vi "Get Remote cRIO Modules Info.vi"(8 "error in":errorcluster, 9 "Device Name":string="RIO0", 10 "cRIO Backplane":T1=enum."cRIO-9068", 11 "IP Address":string) -> (0 "error out":errorcluster, 2 "cRIO Modules":T2[](array[typedef]) {"Serial Number" format="%.0x"; "Vendor and Module ID" format="%.0x"})   [LabVIEW 2015]
uses:
  Controls/cRIO Module Info.ctl
  RT Management/Controls/cRIO Backplanes.ctl
  <vilib>/FPGAPlugInAG/Dynamic/niLvFpga_Run_Dynamic.vi
  <vilib>/FPGAPlugInAG/Dynamic/niLvFpga_Close_Dynamic.vi
  <vilib>/rvi/interface/nirviMethod/nirviMethod.xnode
  <vilib>/rvi/interface/nirviCloseFPGA/nirviCloseFPGA.xnode
  Module Detection.lvclass
  RT Management/RT Management.lvclass
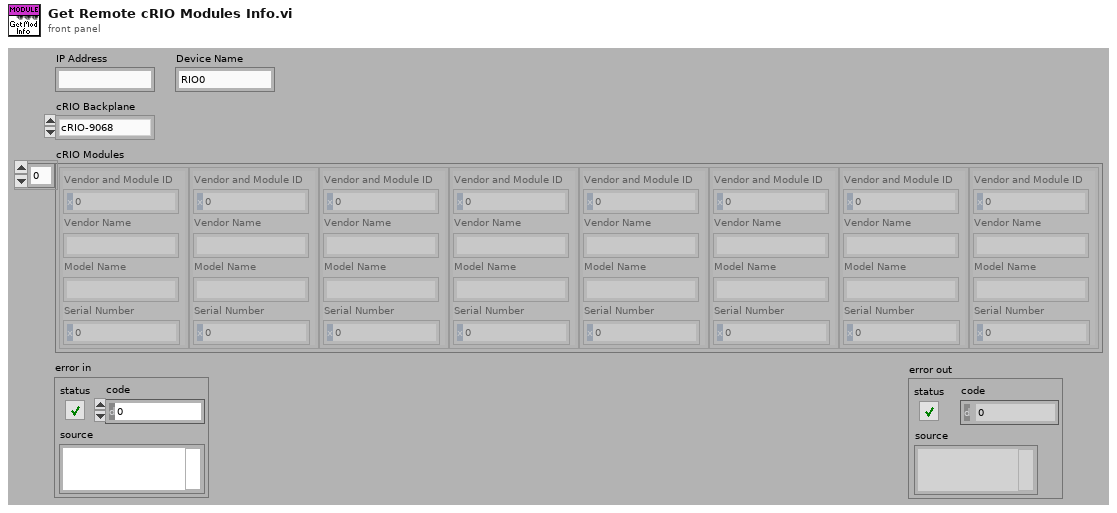
[diagram p1: front panel]
types:
  T1 = typedef "RT Management.lvlib/RT Management.lvclass/cRIO Backplanes.ctl" = enum16{"<Undefined>", "cRIO-9030", "cRIO-9031", "cRIO-9033", "cRIO-9034", "cRIO-9035", "cRIO-9036", "cRIO-9038", "cRIO-9039", "cRIO-9063", "cRIO-9064", "cRIO-9065", "cRIO-9066", "cRIO-9067", "cRIO-9068", "cRIO-9072", "cRIO-9073", "cRIO-9074", "cRIO-9075", "cRIO-9076", "cRIO-9081", "cRIO-9082", "cRIO-9101", "cRIO-9102", "cRIO-9103", "cRIO-9104", "cRIO-9111", "cRIO-9112", "cRIO-9113", "cRIO-9114", "cRIO-9116", "cRIO-9118", "NI 9146", "NI 9147", "NI 9148", "NI 9149", "NI 9154", "NI 9155", "NI 9157", "NI 9159", "myRIO-1900", "myRIO-1950", "sbRIO-9601", "sbRIO-9602", "sbRIO-9605", "sbRIO-9606", "sbRIO-9611", "sbRIO-9612", "sbRIO-9623", "sbRIO-9626", "sbRIO-9631", "sbRIO-9632", "sbRIO-9633", "sbRIO-9636", "sbRIO-9641", "sbRIO-9642"}
  T2 = typedef "RT Management.lvlib/Module Detection.lvclass/cRIO Module Info.ctl" = cluster{"Vendor and Module ID":u32, "Vendor Name":string, "Model Name":string, "Serial Number":u32}
  T3 = cluster{"Vendor and Module ID":u32, "Vendor Name":string, "Model Name":string, "Serial Number":u32}
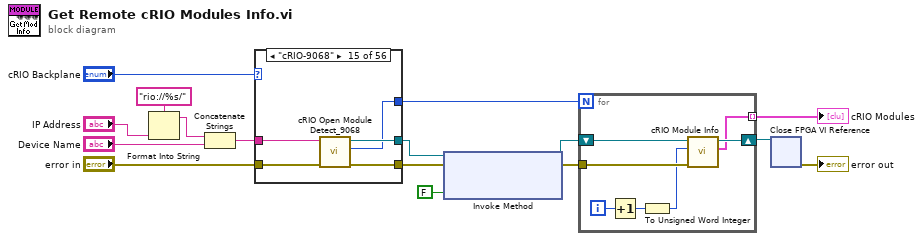
[diagram p0: block diagram]
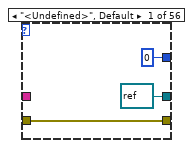
[diagram p2: hidden frame]
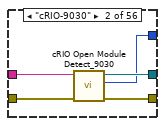
[diagram p3: hidden frame]
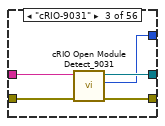
[diagram p4: hidden frame]
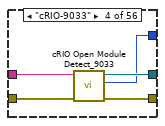
[diagram p5: hidden frame]
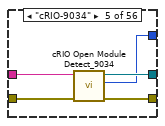
[diagram p6: hidden frame]
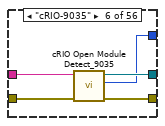
[diagram p7: hidden frame]
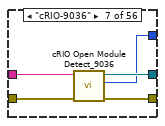
[diagram p8: hidden frame]
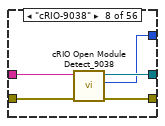
[diagram p9: hidden frame]
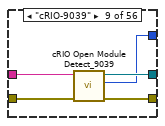
[diagram p10: hidden frame]
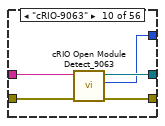
[diagram p11: hidden frame]
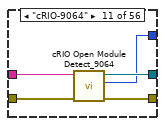
[diagram p12: hidden frame]
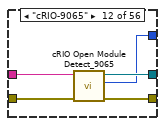
[diagram p13: hidden frame]
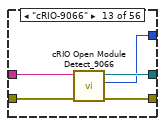
[diagram p14: hidden frame]
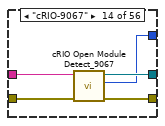
[diagram p15: hidden frame]
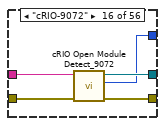
[diagram p16: hidden frame]
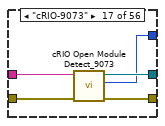
[diagram p17: hidden frame]
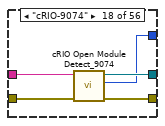
[diagram p18: hidden frame]
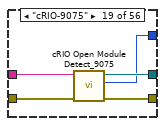
[diagram p19: hidden frame]
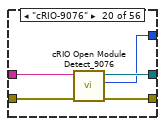
[diagram p20: hidden frame]
diagram:
  n1 = Format Into String(format string="rio://%s/", "IP Address") -> (resulting string=w3:string)  [unwired: 2 in, 1 out]
  n2 = Concatenate Strings(w3, "Device Name") -> (w1:string)
  n3 = case shown="\"cRIO-9068\"" "cRIO Backplane" {
    tunnel: "error in" -> [w19 w23 w28 w33 w38 w43 w48 w53 w58 w63 w68 w73 w78 w83 w88 w93 w98 w103 w108 w113 w118 w123 w128 w133 w138 w143 w148 w153 w158 w164 w169 w174 w179 w184 w189 w194 w199 w204 w209 w214 w217 w220 w225 w230 w233 w236 w241 w246 w249 w252 w257 w262 w265 w268 w273 w278]
    tunnel: [refnum<k20> refnum ("Refnum out") w22 w27 w32 w37 w42 w47 w52 w57 w62 w67 w72 w77 w82 w87 w92 w97 w102 w107 w112 w117 w122 w127 w132 w137 w142 w147 w152 w157 w163 w168 w173 w178 w183 w188 w193 w198 w203 w208 w213 refnum<k20> refnum ("Refnum out") refnum<k20> refnum ("Refnum out") w224 w229 refnum<k20> refnum ("Refnum out") refnum<k20> refnum ("Refnum out") w240 w245 refnum<k20> refnum ("Refnum out") refnum<k20> refnum ("Refnum out") w256 w261 refnum<k20> refnum ("Refnum out") refnum<k20> refnum ("Refnum out") w272 w277] -> w9
    tunnel: [w19 w24 w29 w34 w39 w44 w49 w54 w59 w64 w69 w74 w79 w84 w89 w94 w99 w104 w109 w114 w119 w124 w129 w134 w139 w144 w149 w154 w159 w162 w167 w172 w177 w182 w187 w192 w197 w202 w207 w212 w217 w220 w223 w228 w233 w236 w239 w244 w249 w252 w255 w260 w265 w268 w271 w276] -> w10
    tunnel: [0 ("slots") w21 w26 w31 w36 w41 w46 w51 w56 w61 w66 w71 w76 w81 w86 w91 w96 w101 w106 w111 w116 w121 w126 w131 w136 w141 w146 w151 w156 w161 w166 w171 w176 w181 w186 w191 w196 w201 w206 w211 0 ("slots") 0 ("slots") w222 w227 0 ("slots") 0 ("slots") w238 w243 0 ("slots") 0 ("slots") w254 w259 0 ("slots") 0 ("slots") w270 w275] -> w11
    tunnel: w1 -> [_ w20 w25 w30 w35 w40 w45 w50 w55 w60 w65 w70 w75 w80 w85 w90 w95 w100 w105 w110 w115 w120 w125 w130 w135 w140 w145 w150 w155 w160 w165 w170 w175 w180 w185 w190 w195 w200 w205 w210 _ _ w221 w226 _ _ w237 w242 _ _ w253 w258 _ _ w269 w274]
    frame "<Undefined>", Default {
    }
    frame "cRIO-9030" {
      n4 = call "cRIO Open Module Detect_9030.vi"("error in (no error)"=w23, "RIO Device"=w20) -> ("error out"=w24:errorcluster, "slots"=w21:i32, "Refnum out"=w22:refnum<k20>)  [unwired: 7 in]
    }
    frame "cRIO-9031" {
      n5 = call "cRIO Open Module Detect_9031.vi"("error in (no error)"=w28, "RIO Device"=w25) -> ("error out"=w29:errorcluster, "slots"=w26:i32, "Refnum out"=w27:refnum<k20>)  [unwired: 7 in]
    }
    frame "cRIO-9033" {
      n6 = call "cRIO Open Module Detect_9033.vi"("error in (no error)"=w33, "RIO Device"=w30) -> ("error out"=w34:errorcluster, "slots"=w31:i32, "Refnum out"=w32:refnum<k20>)  [unwired: 7 in]
    }
    frame "cRIO-9034" {
      n7 = call "cRIO Open Module Detect_9034.vi"("error in (no error)"=w38, "RIO Device"=w35) -> ("error out"=w39:errorcluster, "slots"=w36:i32, "Refnum out"=w37:refnum<k20>)  [unwired: 7 in]
    }
    frame "cRIO-9035" {
      n8 = call "cRIO Open Module Detect_9035.vi"("error in"=w43, "RIO Device"=w40) -> ("error out"=w44:errorcluster, "slots"=w41:i32, "Refnum out"=w42:refnum<k20>)  [unwired: 7 in]
    }
    frame "cRIO-9036" {
      n9 = call "cRIO Open Module Detect_9036.vi"("error in"=w48, "RIO Device"=w45) -> ("error out"=w49:errorcluster, "slots"=w46:i32, "Refnum out"=w47:refnum<k20>)  [unwired: 7 in]
    }
    frame "cRIO-9038" {
      n10 = call "cRIO Open Module Detect_9038.vi"("error in (no error)"=w53, "RIO Device"=w50) -> ("error out"=w54:errorcluster, "slots"=w51:i32, "Refnum out"=w52:refnum<k20>)  [unwired: 7 in]
    }
    frame "cRIO-9039" {
      n11 = call "cRIO Open Module Detect_9039.vi"("error in"=w58, "RIO Device"=w55) -> ("error out"=w59:errorcluster, "slots"=w56:i32, "Refnum out"=w57:refnum<k20>)  [unwired: 7 in]
    }
    frame "cRIO-9063" {
      n12 = call "cRIO Open Module Detect_9063.vi"("error in"=w63, "RIO Device"=w60) -> ("error out"=w64:errorcluster, "slots"=w61:i32, "Refnum out"=w62:refnum<k20>)  [unwired: 7 in]
    }
    frame "cRIO-9064" {
      n13 = call "cRIO Open Module Detect_9064.vi"("error in"=w68, "RIO Device"=w65) -> ("error out"=w69:errorcluster, "slots"=w66:i32, "Refnum out"=w67:refnum<k20>)  [unwired: 7 in]
    }
    frame "cRIO-9065" {
      n14 = call "cRIO Open Module Detect_9065.vi"("error in"=w73, "RIO Device"=w70) -> ("error out"=w74:errorcluster, "slots"=w71:i32, "Refnum out"=w72:refnum<k20>)  [unwired: 7 in]
    }
    frame "cRIO-9066" {
      n15 = call "cRIO Open Module Detect_9066.vi"("error in (no error)"=w78, "RIO Device"=w75) -> ("error out"=w79:errorcluster, "slots"=w76:i32, "Refnum out"=w77:refnum<k20>)  [unwired: 7 in]
    }
    frame "cRIO-9067" {
      n16 = call "cRIO Open Module Detect_9067.vi"("error in (no error)"=w83, "RIO Device"=w80) -> ("error out"=w84:errorcluster, "slots"=w81:i32, "Refnum out"=w82:refnum<k20>)  [unwired: 7 in]
    }
    frame "cRIO-9068" {
      n17 = call "cRIO Open Module Detect_9068.vi"("error in"=w88, "RIO Device"=w85) -> ("error out"=w89:errorcluster, "slots"=w86:i32, "Refnum out"=w87:refnum<k20>)  [unwired: 7 in]
    }
    frame "cRIO-9072" {
      n18 = call "cRIO Open Module Detect_9072.vi"("error in (no error)"=w93, "RIO Device"=w90) -> ("error out"=w94:errorcluster, "slots"=w91:i32, "Refnum out"=w92:refnum<k20>)  [unwired: 7 in]
    }
    frame "cRIO-9073" {
      n19 = call "cRIO Open Module Detect_9073.vi"("error in (no error)"=w98, "RIO Device"=w95) -> ("error out"=w99:errorcluster, "slots"=w96:i32, "Refnum out"=w97:refnum<k20>)  [unwired: 7 in]
    }
    frame "cRIO-9074" {
      n20 = call "cRIO Open Module Detect_9074.vi"("error in (no error)"=w103, "RIO Device"=w100) -> ("error out"=w104:errorcluster, "slots"=w101:i32, "Refnum out"=w102:refnum<k20>)  [unwired: 7 in]
    }
    frame "cRIO-9075" {
      n21 = call "cRIO Open Module Detect_9075.vi"("error in (no error)"=w108, "RIO Device"=w105) -> ("error out"=w109:errorcluster, "slots"=w106:i32, "Refnum out"=w107:refnum<k20>)  [unwired: 7 in]
    }
    frame "cRIO-9076" {
      n22 = call "cRIO Open Module Detect_9076.vi"("error in (no error)"=w113, "RIO Device"=w110) -> ("error out"=w114:errorcluster, "slots"=w111:i32, "Refnum out"=w112:refnum<k20>)  [unwired: 7 in]
    }
    frame "cRIO-9081" {
      n23 = call "cRIO Open Module Detect_9081.vi"("error in (no error)"=w118, "RIO Device"=w115) -> ("error out"=w119:errorcluster, "slots"=w116:i32, "Refnum out"=w117:refnum<k20>)  [unwired: 7 in]
    }
    frame "cRIO-9082" {
      n24 = call "cRIO Open Module Detect_9082.vi"("error in (no error)"=w123, "RIO Device"=w120) -> ("error out"=w124:errorcluster, "slots"=w121:i32, "Refnum out"=w122:refnum<k20>)  [unwired: 7 in]
    }
    frame "cRIO-9101" {
      n25 = call "cRIO Open Module Detect_9101.vi"("error in (no error)"=w128, "RIO Device"=w125) -> ("error out"=w129:errorcluster, "slots"=w126:i32, "Refnum out"=w127:refnum<k20>)  [unwired: 7 in]
    }
    frame "cRIO-9102" {
      n26 = call "cRIO Open Module Detect_9102.vi"("error in (no error)"=w133, "RIO Device"=w130) -> ("error out"=w134:errorcluster, "slots"=w131:i32, "Refnum out"=w132:refnum<k20>)  [unwired: 7 in]
    }
    frame "cRIO-9103" {
      n27 = call "cRIO Open Module Detect_9103.vi"("error in (no error)"=w138, "RIO Device"=w135) -> ("error out"=w139:errorcluster, "slots"=w136:i32, "Refnum out"=w137:refnum<k20>)  [unwired: 7 in]
    }
    frame "cRIO-9104" {
      n28 = call "cRIO Open Module Detect_9104.vi"("error in (no error)"=w143, "RIO Device"=w140) -> ("error out"=w144:errorcluster, "slots"=w141:i32, "Refnum out"=w142:refnum<k20>)  [unwired: 7 in]
    }
    frame "cRIO-9111" {
      n29 = call "cRIO Open Module Detect_9111.vi"("error in (no error)"=w148, "RIO Device"=w145) -> ("error out"=w149:errorcluster, "slots"=w146:i32, "Refnum out"=w147:refnum<k20>)  [unwired: 7 in]
    }
    frame "cRIO-9112" {
      n30 = call "cRIO Open Module Detect_9112.vi"("error in (no error)"=w153, "RIO Device"=w150) -> ("error out"=w154:errorcluster, "slots"=w151:i32, "Refnum out"=w152:refnum<k20>)  [unwired: 7 in]
    }
    frame "cRIO-9113" {
      n31 = call "cRIO Open Module Detect_9113.vi"("error in (no error)"=w158, "RIO Device"=w155) -> ("error out"=w159:errorcluster, "slots"=w156:i32, "Refnum out"=w157:refnum<k20>)  [unwired: 7 in]
    }
    frame "cRIO-9114" {
      n32 = call "cRIO Open Module Detect_9114.vi"("error in (no error)"=w164, "RIO Device"=w160) -> ("error out"=w162:errorcluster, "slots"=w161:i32, "Refnum out"=w163:refnum<k20>)  [unwired: 7 in]
    }
    frame "cRIO-9116" {
      n33 = call "cRIO Open Module Detect_9116.vi"("error in (no error)"=w169, "RIO Device"=w165) -> ("error out"=w167:errorcluster, "slots"=w166:i32, "Refnum out"=w168:refnum<k20>)  [unwired: 7 in]
    }
    frame "cRIO-9118" {
      n34 = call "cRIO Open Module Detect_9118.vi"("error in (no error)"=w174, "RIO Device"=w170) -> ("error out"=w172:errorcluster, "slots"=w171:i32, "Refnum out"=w173:refnum<k20>)  [unwired: 7 in]
    }
    frame "NI 9146" {
      n35 = call "Ethernet RIO Open Module Detect_9146.vi"("error in"=w179, "RIO Device"=w175) -> ("error out"=w177:errorcluster, "slots"=w176:i32, "Refnum out"=w178:refnum<k20>)  [unwired: 7 in]
    }
    frame "NI 9147" {
      n36 = call "Ethernet RIO Open Module Detect_9147.vi"("error in (no error)"=w184, "RIO Device"=w180) -> ("error out"=w182:errorcluster, "slots"=w181:i32, "Refnum out"=w183:refnum<k20>)  [unwired: 7 in]
    }
    frame "NI 9148" {
      n37 = call "Ethernet RIO Open Module Detect_9148.vi"("error in (no error)"=w189, "RIO Device"=w185) -> ("error out"=w187:errorcluster, "slots"=w186:i32, "Refnum out"=w188:refnum<k20>)  [unwired: 7 in]
    }
    frame "NI 9149" {
      n38 = call "Ethernet RIO Open Module Detect_9149.vi"("error in (no error)"=w194, "RIO Device"=w190) -> ("error out"=w192:errorcluster, "slots"=w191:i32, "Refnum out"=w193:refnum<k20>)  [unwired: 7 in]
    }
    frame "NI 9154" {
      n39 = call "MXI-Express RIO Open Module Detect_9154.vi"("error in"=w199, "RIO Device"=w195) -> ("error out"=w197:errorcluster, "slots"=w196:i32, "Refnum out"=w198:refnum<k20>)  [unwired: 7 in]
    }
    frame "NI 9155" {
      n40 = call "MXI-Express RIO Open Module Detect_9155.vi"("error in"=w204, "RIO Device"=w200) -> ("error out"=w202:errorcluster, "slots"=w201:i32, "Refnum out"=w203:refnum<k20>)  [unwired: 7 in]
    }
    frame "NI 9157" {
      n41 = call "MXI-Express RIO Open Module Detect_9157.vi"("error in (no error)"=w209, "RIO Device"=w205) -> ("error out"=w207:errorcluster, "slots"=w206:i32, "Refnum out"=w208:refnum<k20>)  [unwired: 7 in]
    }
    frame "NI 9159" {
      n42 = call "MXI-Express RIO Open Module Detect_9159.vi"("error in (no error)"=w214, "RIO Device"=w210) -> ("error out"=w212:errorcluster, "slots"=w211:i32, "Refnum out"=w213:refnum<k20>)  [unwired: 7 in]
    }
    frame "myRIO-1900" {
    }
    frame "myRIO-1950" {
    }
    frame "sbRIO-9601" {
      n43 = call "sbRIO Open Module Detect_9601.vi"("error in (no error)"=w225, "RIO Device"=w221) -> ("error out"=w223:errorcluster, "slots"=w222:i32, "Refnum out"=w224:refnum<k20>)  [unwired: 7 in]
    }
    frame "sbRIO-9602" {
      n44 = call "sbRIO Open Module Detect_9602.vi"("error in (no error)"=w230, "RIO Device"=w226) -> ("error out"=w228:errorcluster, "slots"=w227:i32, "Refnum out"=w229:refnum<k20>)  [unwired: 7 in]
    }
    frame "sbRIO-9605" {
    }
    frame "sbRIO-9606" {
    }
    frame "sbRIO-9611" {
      n45 = call "sbRIO Open Module Detect_9611.vi"("error in"=w241, "RIO Device"=w237) -> ("error out"=w239:errorcluster, "slots"=w238:i32, "Refnum out"=w240:refnum<k20>)  [unwired: 7 in]
    }
    frame "sbRIO-9612" {
      n46 = call "sbRIO Open Module Detect_9612.vi"("error in"=w246, "RIO Device"=w242) -> ("error out"=w244:errorcluster, "slots"=w243:i32, "Refnum out"=w245:refnum<k20>)  [unwired: 7 in]
    }
    frame "sbRIO-9623" {
    }
    frame "sbRIO-9626" {
    }
    frame "sbRIO-9631" {
      n47 = call "sbRIO Open Module Detect_9631.vi"("error in"=w257, "RIO Device"=w253) -> ("error out"=w255:errorcluster, "slots"=w254:i32, "Refnum out"=w256:refnum<k20>)  [unwired: 7 in]
    }
    frame "sbRIO-9632" {
      n48 = call "sbRIO Open Module Detect_9632.vi"("error in"=w262, "RIO Device"=w258) -> ("error out"=w260:errorcluster, "slots"=w259:i32, "Refnum out"=w261:refnum<k20>)  [unwired: 7 in]
    }
    frame "sbRIO-9633" {
    }
    frame "sbRIO-9636" {
    }
    frame "sbRIO-9641" {
      n49 = call "sbRIO Open Module Detect_9641.vi"("error in"=w273, "RIO Device"=w269) -> ("error out"=w271:errorcluster, "slots"=w270:i32, "Refnum out"=w272:refnum<k20>)  [unwired: 7 in]
    }
    frame "sbRIO-9642" {
      n50 = call "sbRIO Open Module Detect_9642.vi"("error in"=w278, "RIO Device"=w274) -> ("error out"=w276:errorcluster, "slots"=w275:i32, "Refnum out"=w277:refnum<k20>)  [unwired: 7 in]
    }
  }
  n51 = xnode "Invoke Method"("FPGA VI Reference In"=w9, "error in"=w10, "Wait Until Done (F)"=FALSE) -> ("FPGA VI Reference Out"=w14:refnum<k20>, "error out"=w13:errorcluster)
  n52 = for {
    N: w11 -> [_]
    shift-right: [w283] -> w12
    shift-left: w14 -> [w285]
    tunnel: [w279] -> w8 mode=indexing
    tunnel: w13 -> [w284]
    i -> [w282]
    n53 = Increment(x=w282) -> (x+1=w281:i32)
    n54 = To Unsigned Word Integer(number=w281) -> (unsigned 16bit integer=w280:u16)
    n55 = call "cRIO Module Info.vi"("error in"=w284, "Module"=w280, "Refnum in"=w285) -> ("cRIO Module Info"=w279:T3, "Refnum out"=w283:refnum<k20>)  [unwired: 6 in, 1 out]
  }
  "cRIO Modules" <- w8
  n56 = xnode "Close FPGA VI Reference"("FPGA VI Reference In"=w12) -> ("error out"=→"error out":errorcluster)  [unwired: 1 in]
